vi "Stop Server.vi"(8 "error in":errorcluster, 11 "gRPC Server in":refnum<class "Servicer.lvclass">) -> (0 "error out":errorcluster)   [LabVIEW 2024, in "gRPC-servicer.lvlib" / "Servicer.lvclass"]
uses:
  Servicer.lvclass
  Servicer.lvclass/Servicer.ctl
  gRPC lv Support/grpc-lvsupport/grpc-lvsupport.lvlib
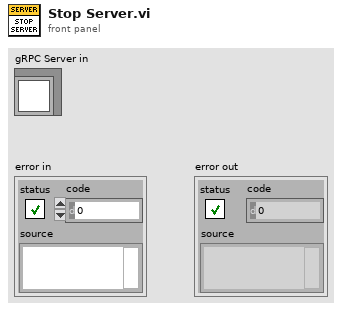
[diagram p1: front panel]
types:
  T1 = typedef "grpc-lvsupport.lvlib/grpcId.ctl" = u64
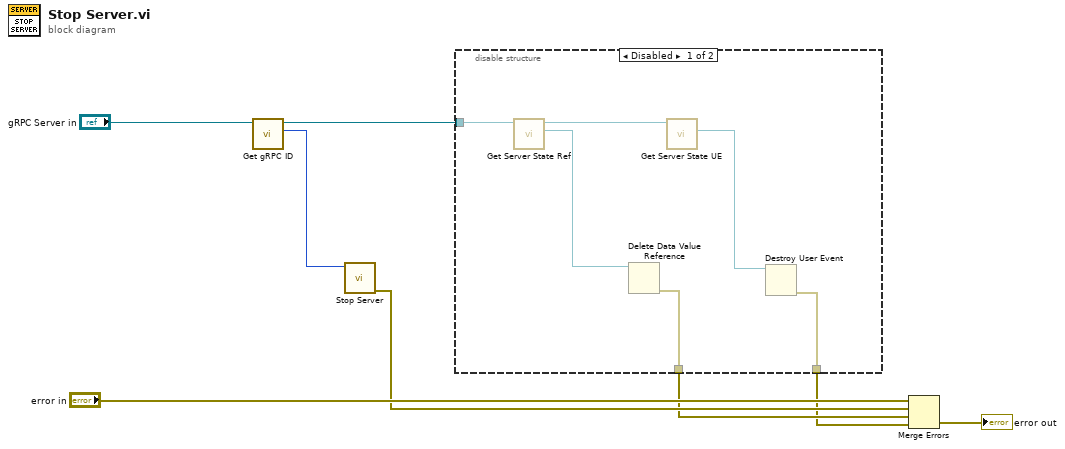
[diagram p0: block diagram]
diagram:
  n1 = call "Get gRPC ID.vi"("OOP Server in"="gRPC Server in") -> ("gRPC ID"=w6:T1, "OOP Server out"=w5:refnum<class "Servicer.lvclass">)  [unwired: 9 in]
  n2 = call "Stop Server.vi"("gRPCid server in"=w6) -> ("error out"=w3:errorcluster)  [unwired: 10 in]
  n3 = disable-structure shown="Disabled" {
    disable-tunnel: w5 -> [w12 _]
    disable-tunnel: [w14 _] -> w2
    disable-tunnel: [w13 _] -> w1
    frame Disabled {
      n4 = call "Get Server State Ref.vi"("Template Server in"=w12) -> ("Server State Ref"=w10:refnum<data-value>, "Template Server out"=w11:refnum<class "Servicer.lvclass">)  [unwired: 9 in]
      n5 = Delete Data Value Reference(data value reference=w10) -> (error out=w14:errorcluster)  [unwired: 1 in, 1 out]
      n6 = call "Get Server State UE.vi"("Template Server in"=w11) -> ("Server Internal State UE"=w9:refnum<user-event>)  [unwired: 9 in, 1 out]
      n7 = Destroy User Event(user event=w9) -> (error out=w13:errorcluster)  [unwired: 1 in]
    }
    frame Enabled {
    }
  }
  n8 = Merge Errors("error in", w3, w2, w1) -> (→"error out":errorcluster)
